vi "insert.vi"(8 "error in (no error)":errorcluster, 10 "To Insert":T1, 11 "Bucket in":refnum<class "Bucket.lvclass">) -> (0 "error out":errorcluster, 3 "Bucket out":refnum<class "Bucket.lvclass">)   [LabVIEW 2017, in "Bucket.lvclass"]
uses:
  <userlib>/836-Library/Data_Structures/HashMap/Support/Bucket/Bucket.lvclass
  <userlib>/836-Library/Data_Structures/HashMap/Support/Bucket/Types/KeyValuePair.ctl
  <userlib>/836-Library/Data_Structures/HashMap/Support/Bucket/Bucket.lvclass/Bucket.ctl
  <vilib>/Utility/error.llb/Error Cluster From Error Code.vi
  <vilib>/ErrorRing/Error Ring.xnode
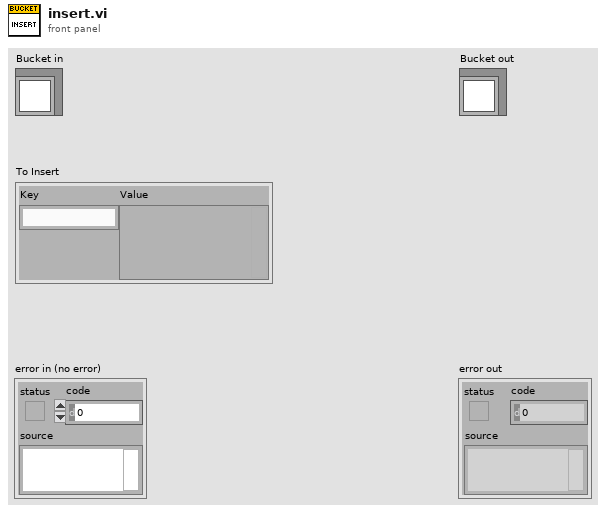
[diagram p1: front panel]
types:
  T1 = typedef "KeyValuePair.ctl" = cluster{"Key":string, "Value":variant}
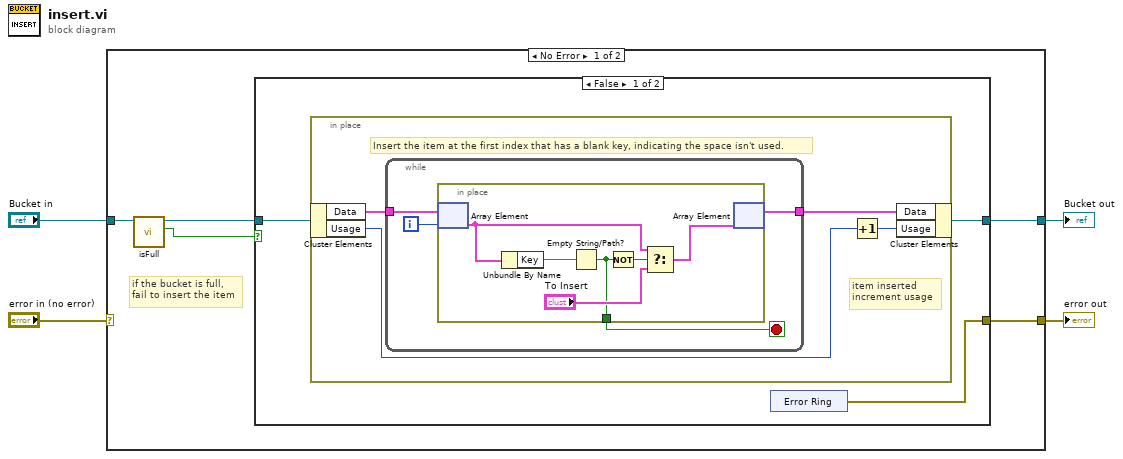
[diagram p0: block diagram]
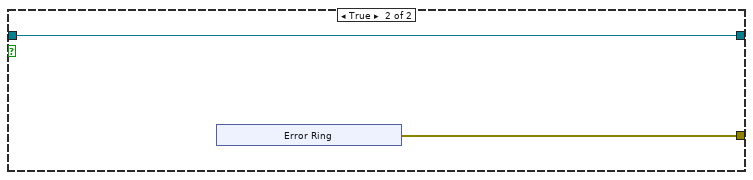
[diagram p2: hidden frame]
diagram:
  n1 = case shown="No Error" "error in (no error)" {
    selector: "error in (no error)" -> [_ w36]
    tunnel: [w5 w36] -> w3
    tunnel: [w6 w35] -> w1
    tunnel: "Bucket in" -> [w9 w35]
    frame No Error {
      # "if the bucket is full,\nfail to insert the item"
      n2 = call <userlib>:"isFull.vi"("Bucket in"=w9) -> ("Full?"=w8:bool, "Bucket out"=w7:refnum<class "Bucket.lvclass">)  [unwired: 8 in, 1 out]
      n3 = case shown="False" w8 {
        tunnel: [w10 w29] -> w5
        tunnel: w7 -> [w12 w28]
        tunnel: [w11 w28] -> w6
        frame False {
          n4 = in-place {
            # "item inserted\nincrement usage"
            # "Insert the item at the first index that has a blank key, indicating the space isn't used."
            n5 = in-place-cluster #1(w12) -> ("Data"=w17:T1[], "Usage"=w14:u32)
            n6 = while {
              tunnel: w17 -> [w21]
              tunnel: [w18] -> w16
              i -> [w20]
              stop <- w19 stop-if-true
              n7 = in-place {
                in-place-border: [w22] -> w19
                n8 = in-place-array #2(w21, w20) -> (w25:T1)
                n9 = Unbundle By Name(w25) -> ("Key"=w27:string)
                n10 = Empty String/Path?(string/path=w27) -> (empty?=w22:bool)
                n11 = Not(x=w22) -> (.not. x?=w26:bool)
                n12 = Select(t=w25, s=w26, f="To Insert") -> (s? t:f=w23:T1)
                n13 = in-place-array #2(w23) -> (w18:T1[])  [unwired: 1 out]
              }
            }
            n14 = Increment(x=w14) -> (x+1=w15:u32)
            n15 = in-place-cluster #1("Data"=w16, "Usage"=w15) -> (w11:refnum<class "Bucket.lvclass">)
          }
          n16 = xnode "Error Ring"() -> ("error out"=w10:errorcluster)
        }
        frame True {
          n17 = xnode "Error Ring"() -> ("error out"=w29:errorcluster)
        }
      }
    }
    frame Error {
    }
  }
  "error out" <- w3
  "Bucket out" <- w1
